vi "Tosca-Visual Display Thread.vi"(0 "IPC":T1) -> (15 "error out":errorcluster)   [LabVIEW 2020]
uses:
  IPC VIs/Tosca-IPC.ctl
  Classes/Parameters/Parameters.lvclass
  Digital Input VIs/Tosca-DI Queue Data.ctl
  Digital Input VIs/Tosca-Input Event.ctl
  Digital Input VIs/Tosca-Input Criterion.ctl
  epl-vi-lib/Utility VIs/Type Defs/Logic State.ctl
  Typedefs/Tosca-Accumulator.ctl
  Typedefs/Tosca-State AODO.ctl
  Typedefs/Tosca-AO Runtime.ctl
  Typedefs/Tosca-DO Runtime.ctl
  epl-vi-lib/Signal Synthesis VIs/4th Generation/Classes/SignalManager/SignalManager.lvclass
  Typedefs/Tosca-Synapse Start Data.ctl
  IPC VIs/Tosca-Message.ctl
  IPC VIs/Tosca-Message Action.ctl
  Typedefs/Tosca-Thread Type.ctl
  Imaging VIs/Tosca-2P-Notifier Data.ctl
  Typedefs/Tosca-MATLAB Queue Data.ctl
  Tosca-Grating.ctl
  Tosca-Grating Type.ctl
  Typedefs/Tosca-File IO Notification.ctl
  Trace VIs/Tosca-Trace-Event.ctl
  Sub VIs/Tosca-Globals.vi
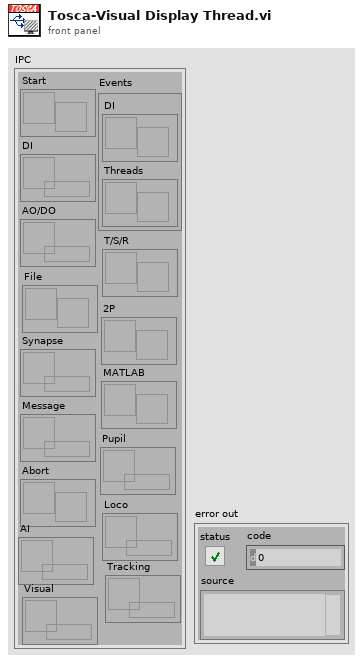
[diagram p1: front panel]
types:
  T1 = typedef "Tosca-IPC.ctl" = cluster{"Start":refnum<notifier>, "DI":refnum<queue>, "AO/DO":refnum<queue>, "Synapse":refnum<queue>, "Message":refnum<queue>, "Abort":refnum<notifier>, "Events":cluster{"DI":refnum<user-event>, "Threads ":refnum<user-event>}, "T/S/R":refnum<notifier>, "2P":refnum<notifier>, "MATLAB":refnum<notifier>, "Pupil":refnum<queue>, "Loco":refnum<queue>, "AI":refnum<queue>, "Tracking":refnum<queue>, "Visual":refnum<queue>, "File":refnum<notifier>}
  T2 = typedef "Tosca-Thread Type.ctl" = enum16{"None", "AODO", "Masker", "ET", "Imaging", "Pupil", "AI", "DI", "Camera", "TTL out", "Loco", "Visual"}
  T3 = typedef "Tosca-Visual Display Settings.ctl" = cluster{"Use PTB":bool, "IP Address":string, "Port":i32, "rect":cluster{"left":i16, "top":i16, "width":i16, "height":i16}, "Full screen":bool, "Open at start":bool, "Monitor":i32, "Monitor size (in)":dbl, "Monitor dist (in)":dbl, "Photodiode Square":cluster{"size":i16, "location":enum16{"Bottom Left", "Top Left", "Top Right", "Bottom Right"}}, "Background":dbl}
  T4 = typedef "Tosca-Trace-Event.ctl" = enum16{"Unspecified", "Trial start", "Enqueue", "Result", "End parser", "Frame", "Queue available", "Timeout sent", "WritePos", "TTL"}
  T5 = typedef "Tosca-Grating.ctl" = cluster{"Type":T6, "Orientation (deg)":dbl, "Spatial frequency (cpd)":dbl, "Velocity (Hz)":dbl, "Contrast":dbl, "Background intensity":dbl, "Duration (ms)":dbl, "Phase (cycles)":dbl}
  T6 = typedef "Tosca-Grating Type.ctl" = enum16{"OFF", "Square", "Sine"}
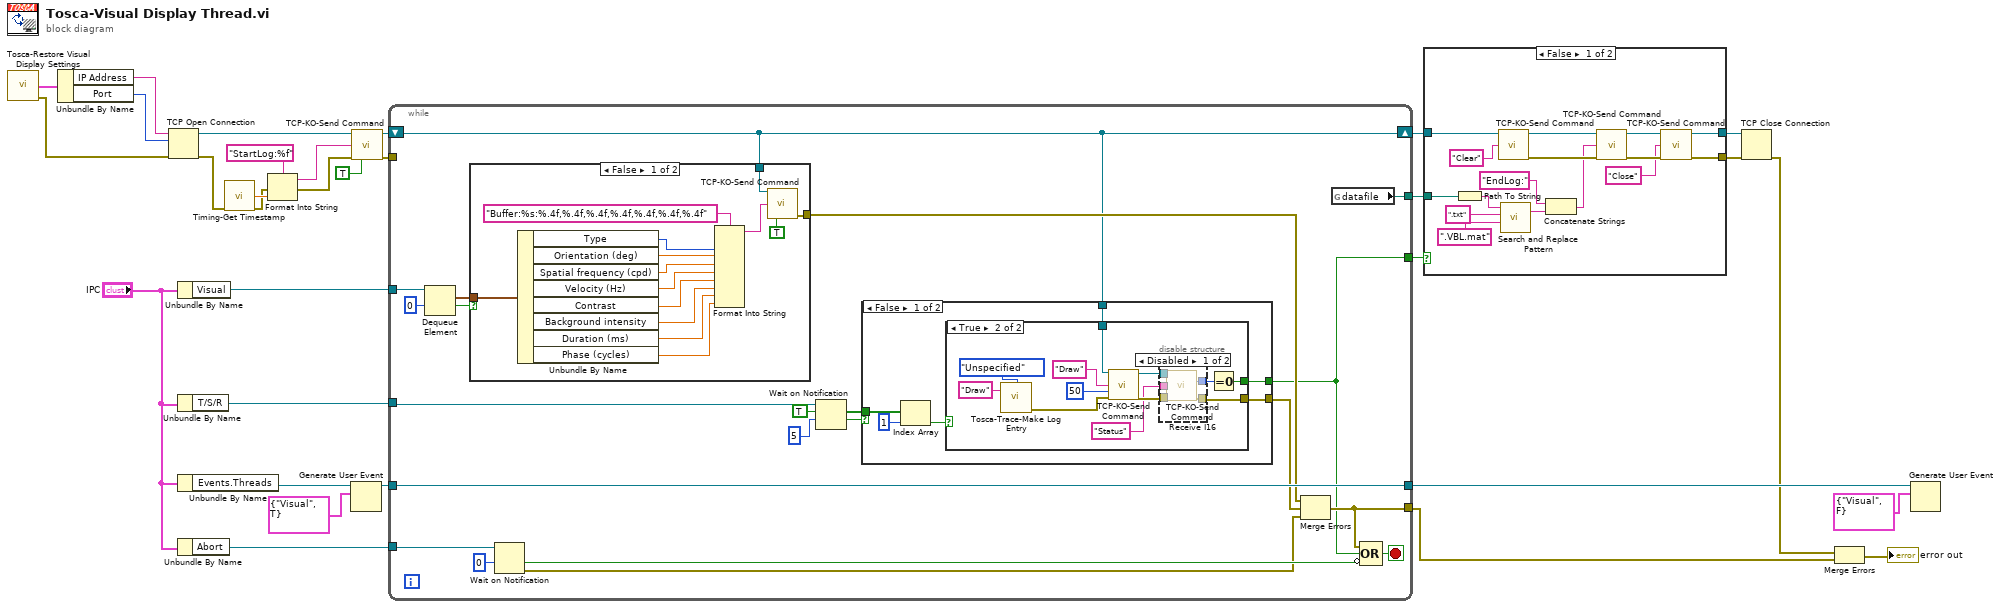
[diagram p0: block diagram]
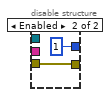
[diagram p4: hidden frame]
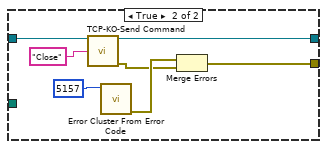
[diagram p6: hidden frame]
diagram:
  n1 = call "Tosca-Restore Visual Display Settings.vi"() -> ("Visual Display Settings"=w21:T3, "error out"=w12:errorcluster)  [unwired: 14 in]
  n2 = Unbundle By Name(w21) -> ("IP Address"=w14:string, "Port"=w13:i32)
  n3 = TCP Open Connection(address=w14, remote port or service name=w13, error in (no error)=w12) -> (connection ID=w11:refnum<k5>, error out=w10:errorcluster)  [unwired: 2 in]
  n4 = Unbundle By Name("IPC") -> ("Visual"=w19:refnum<queue>)
  n5 = Unbundle By Name("IPC") -> ("T/S/R"=w22:refnum<notifier>)
  n6 = Unbundle By Name("IPC") -> ("Events.Threads"=w31:refnum<user-event>)
  n7 = Unbundle By Name("IPC") -> ("Abort"=w26:refnum<notifier>)
  n8 = call "Timing-Get Timestamp.vi"("error in (no error)"=w10) -> ("double precision float"=w17:dbl, "error out"=w16:errorcluster)  [unwired: 13 in]
  n9 = Format Into String(format string="StartLog:%f", error in=w16, w17) -> (resulting string=w9:string, error out=w8:errorcluster)  [unwired: 1 in]
  n10 = Generate User Event(user event=w31, event data cluster=cluster{"ID":T2, "Running":bool} {"ID"=enum."Visual", "Running"=TRUE} ("event data")) -> (user event out=w29:refnum<user-event>)  [unwired: 2 in, 1 out]
  n11 = call "TCP-KO-Send Command.vi"("connection ID"=w11, "Command"=w9, "error in (no error)"=w8, "fast response"=TRUE) -> ("connection ID out"=w5:refnum<k5>, "error out"=w6:errorcluster)  [unwired: 10 in]
  n12 = while {
    tunnel: w29 -> [w52]
    tunnel: [w52] -> w28
    tunnel: w26 -> [w49]
    tunnel: [w34] -> w24
    tunnel: [w46] -> w23
    tunnel: w22 -> [w43]
    tunnel: w19 -> [w39]
    tunnel: [w33] -> w15
    tunnel: w6 -> [_]
    shift-right: [w32] -> w4
    shift-left: w5 -> [w32]
    stop <- w48 stop-if-true
    n13 = Dequeue Element(queue=w39, timeout in ms (-1)=0) -> (element=w36:T5, timed out?=w37:bool)  [unwired: 1 in, 2 out]
    n14 = case shown="False" w37 {
      tunnel: w36 -> [w58 _]
      tunnel: [w53 _] -> w35
      tunnel: w32 -> [w56 _]
      frame False {
        n15 = Unbundle By Name(w58) -> ("Type"=w60:T6, "Orientation (deg)"=w61:dbl, "Spatial frequency (cpd)"=w62:dbl, "Velocity (Hz)"=w63:dbl, "Contrast"=w64:dbl, "Background intensity"=w65:dbl, "Duration (ms)"=w66:dbl, "Phase (cycles)"=w57:dbl)
        n16 = Format Into String(format string="Buffer:%s:%.4f,%.4f,%.4f,%.4f,%.4f,%.4f,%.4f", w60, w61, w62, w63, w64, w65, w66, w57) -> (resulting string=w54:string)  [unwired: 2 in, 1 out]
        n17 = call "TCP-KO-Send Command.vi"("connection ID"=w56, "Command"=w54, "fast response"=TRUE) -> ("error out"=w53:errorcluster)  [unwired: 11 in, 1 out]
      }
      frame True {
      }
    }
    n18 = Wait on Notification(notifier=w49, timeout in ms (-1)=0) -> (timed out?=w51:bool, error out=w47:errorcluster)  [unwired: 2 in, 2 out]
    n19 = Wait on Notification(notifier=w43, ignore previous (F)=TRUE, timeout in ms (-1)=5) -> (notification=w41:bool[], timed out?=w42:bool)  [unwired: 1 in, 2 out]
    n20 = case shown="False" w42 {
      tunnel: w41 -> [w71 _]
      tunnel: [w70 _] -> w40
      tunnel: [w68 _] -> w34
      tunnel: w32 -> [w67 _]
      frame False {
        n21 = Index Array(array=w71, index=1) -> (element=w72:bool)
        n22 = case shown="True" w72 {
          tunnel: [_ w78] -> w70
          tunnel: [_ w84] -> w68
          tunnel: w67 -> [_ w79]
          frame False {
          }
          frame True {
            n23 = call "Tosca-Trace-Make Log Entry.vi"("Message"="Draw", "Event"=Tosca-Trace-Event."Unspecified") -> ("error out"=w80:errorcluster)  [unwired: 13 in]
            n24 = call "TCP-KO-Send Command.vi"("connection ID"=w79, "Command"="Draw" ("format string"), "timeout (ms)"=50, "error in (no error)"=w80) -> ("connection ID out"=w75:refnum<k5>, "error out"=w76:errorcluster)  [unwired: 10 in]
            n25 = disable-structure shown="Disabled" {
              disable-tunnel: [w89 w91] -> w78
              disable-tunnel: [w88 i16 1 ("value")] -> w77
              disable-tunnel: w76 -> [w87 w91]
              disable-tunnel: w75 -> [w86 _]
              disable-tunnel: "Status" ("Command") -> [w85 _]
              frame Disabled {
                n26 = call "TCP-KO-Send Command Receive I16.vi"("connection ID"=w86, "Command"=w85, "error in (no error)"=w87) -> ("value"=w88:i16, "error out"=w89:errorcluster)  [unwired: 9 in, 2 out]
              }
              frame Enabled {
              }
            }
            n27 = Equal To 0?(x=w77) -> (x = 0?=w84:bool)
          }
        }
      }
      frame True {
      }
    }
    n28 = Merge Errors(w35, w40, w47) -> (w46:errorcluster)
    n29 = global read "Tosca-Globals.vi" "datafile"() -> (w33:path)
    n30 = Compound Arithmetic op=OR(w46, w34, invert w51) -> (w48:bool)
  }
  n31 = case shown="False" w24 {
    tunnel: [w93 w110] -> w3
    tunnel: w15 -> [w102 _]
    tunnel: w4 -> [w100 w112]
    tunnel: [w92 w108] -> w2
    frame False {
      n32 = Path To String(path=w102) -> (string=w103:string)
      n33 = call "TCP-KO-Send Command.vi"("connection ID"=w100, "Command"="Clear") -> ("connection ID out"=w98:refnum<k5>, "error out"=w99:errorcluster)  [unwired: 12 in]
      n34 = call <vilib>:"Search and Replace Pattern.vi"("string"=w103, "regular expression (\"\")"=".txt" ("regular expression (\"\")"), "replace string (\"\")"=".VBL.mat" ("replace string (\"\")")) -> ("result string"=w106:string)  [unwired: 2 in, 1 out]
      n35 = Concatenate Strings("EndLog:" ("Command"), w106) -> (w97:string)
      n36 = call "TCP-KO-Send Command.vi"("connection ID"=w98, "Command"=w97, "error in (no error)"=w99) -> ("connection ID out"=w96:refnum<k5>, "error out"=w95:errorcluster)  [unwired: 11 in]
      n37 = call "TCP-KO-Send Command.vi"("connection ID"=w96, "Command"="Close", "error in (no error)"=w95) -> ("connection ID out"=w92:refnum<k5>, "error out"=w93:errorcluster)  [unwired: 11 in]
    }
    frame True {
      n38 = call "TCP-KO-Send Command.vi"("connection ID"=w112, "Command"="Close") -> ("connection ID out"=w108:refnum<k5>, "error out"=w109:errorcluster)  [unwired: 12 in]
      n39 = call <vilib>:"Error Cluster From Error Code.vi"("error code (0)"=5157) -> ("error out"=w113:errorcluster)  [unwired: 8 in]
      n40 = Merge Errors(w113, w109) -> (w110:errorcluster)
    }
  }
  n41 = TCP Close Connection(connection ID=w2, error in (no error)=w3) -> (error out=w1:errorcluster)  [unwired: 1 in, 1 out]
  n42 = Merge Errors(w1, w23) -> (→"error out":errorcluster)
  n43 = Generate User Event(user event=w28, event data cluster=cluster{"ID":T2, "Running":bool} {"ID"=enum."Visual", "Running"=FALSE} ("event data")) -> ()  [unwired: 2 in, 2 out]
